vi "Access DB Path.vi"(9 "Password":string, 10 "ping":bool, 11 "database":string="database1.mdb") -> (2 "Connection information":string, 3 "Path out":string)   [LabVIEW 2016, in "Access Lib.lvlib"]
uses:
  Access Lib.lvlib
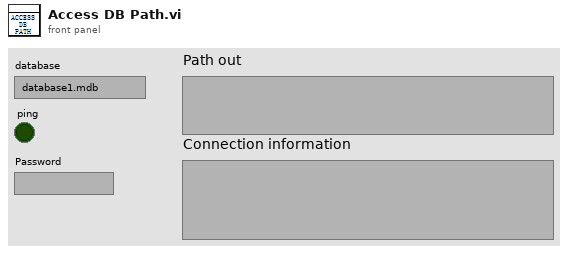
[diagram p1: front panel]
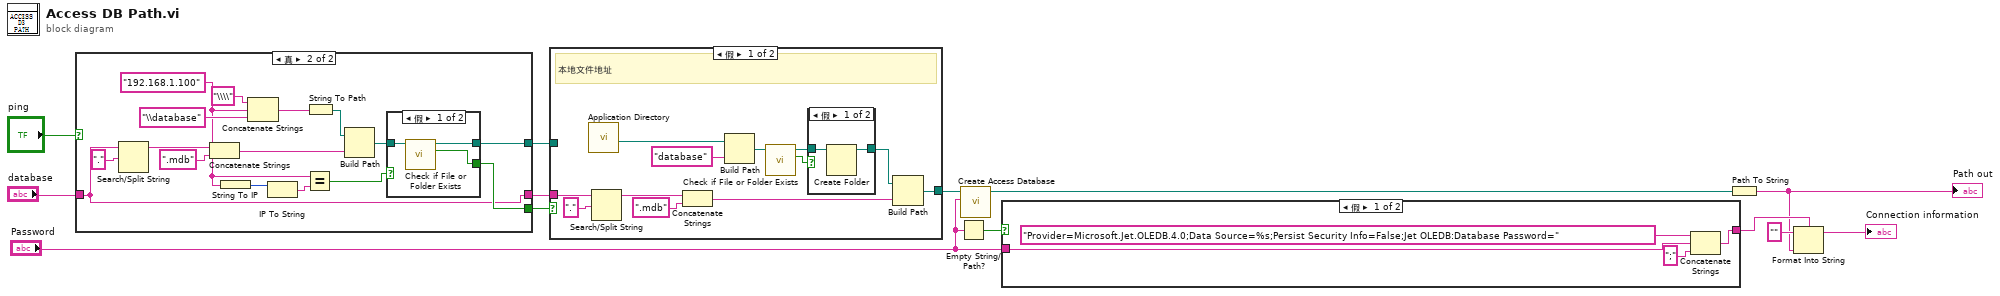
[diagram p0: block diagram]
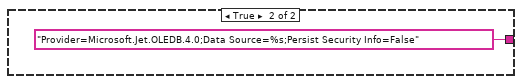
[diagram p2: hidden frame]
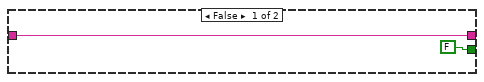
[diagram p5: hidden frame]
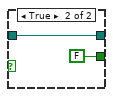
[diagram p6: hidden frame]
diagram:
  n1 = case shown="真" "ping" {
    tunnel: [_ w25] -> w9
    tunnel: [FALSE ("file or folder exists?") w24] -> w10
    tunnel: [w14 w19] -> w11
    tunnel: "database" -> [w14 w19]
    frame False {
    }
    frame True {
      w16 = "192.168.1.100" ("名称")
      n2 = Search/Split String(string=w19, search string/char (-)="." ("搜索字符串/字符(-)")) -> (substring before match=w23:string)  [unwired: 1 in, 2 out]
      n3 = Concatenate Strings(w23, ".mdb" ("字符串")) -> (w20:string)
      n4 = String To IP(1:w16) -> (0:w31:u32)
      n5 = Concatenate Strings("\\\\" ("字符串"), w16, "\\database" ("名称或相对路径")) -> (w29:string)
      n6 = IP To String(2:w31) -> (0:w28:string)  [unwired: 1 in]
      n7 = Equal?(x=w16, y=w28) -> (x = y?=w27:bool)
      n8 = String To Path(string=w29) -> (path=w18:path)
      n9 = Build Path(base path=w18, name or relative path=w20) -> (appended path=w26:path)
      n10 = case shown="假" w27 {
        tunnel: w26 -> [w34 w35]
        tunnel: [w33 w35] -> w25
        tunnel: [w32 FALSE] -> w24
        frame False {
          n11 = call <vilib>:"Check if File or Folder Exists.vi"("path"=w34) -> ("file or folder exists?"=w32:bool, "dup path"=w33:path)  [unwired: 8 in, 1 out]
        }
        frame True {
        }
      }
    }
  }
  n12 = case shown="假" w10 {
    tunnel: w11 -> [w40 _]
    tunnel: [w38 w52] -> w13
    tunnel: w9 -> [_ w52]
    frame False {
      # "本地文件地址"
      n13 = call <vilib>:"Application Directory.vi"() -> ("Application Directory"=w37:path)
      n14 = Search/Split String(string=w40, search string/char (-)="." ("搜索字符串/字符(-)")) -> (substring before match=w43:string)  [unwired: 1 in, 2 out]
      n15 = Concatenate Strings(w43, ".mdb" ("字符串")) -> (w39:string)
      n16 = Build Path(base path=w37, name or relative path="database" ("名称或相对路径")) -> (appended path=w44:path)
      n17 = call <vilib>:"Check if File or Folder Exists.vi"("path"=w44) -> ("file or folder exists?"=w48:bool, "dup path"=w47:path)  [unwired: 8 in, 1 out]
      n18 = case shown="假" w48 {
        tunnel: w47 -> [w50 w51]
        tunnel: [w49 w51] -> w46
        frame False {
          n19 = Create Folder(path (use dialog)=w50) -> (created path=w49:path)  [unwired: 2 in, 2 out]
        }
        frame True {
        }
      }
      n20 = Build Path(base path=w46, name or relative path=w39) -> (appended path=w38:path)
    }
    frame True {
      # "共享文件地址"
    }
  }
  n21 = Empty String/Path?(string/path="Password") -> (empty?=w6:bool)
  n22 = call "Create Access Database.vi"("Password"="Password", "路径"=w13) -> ("路径 out"=w7:path)  [unwired: 8 in, 1 out]
  n23 = case shown="假" w6 {
    tunnel: [w53 "Provider=Microsoft.Jet.OLEDB.4.0;Data Source=%s;Persist Security Info=False" ("格式字符串")] -> w4
    tunnel: "Password" -> [w56 _]
    frame False {
      n24 = Concatenate Strings("Provider=Microsoft.Jet.OLEDB.4.0;Data Source=%s;Persist Security Info=False;Jet OLEDB:Database Password=" ("格式字符串"), w56, ";" ("字符串")) -> (w53:string)
    }
    frame True {
    }
  }
  n25 = Path To String(path=w7) -> (string=w2:string)
  "Path out" <- w2
  n26 = Format Into String(format string=w4, initial string="" ("初始字符串"), w2) -> (resulting string=→"Connection information":string)  [unwired: 1 in, 1 out]
